vi "Img Load Frame Pic.vi"(8 "error in (no error)":errorcluster, 9 "Rectangle":T1, 10 "Image Path":path, 11 "Image In":T2) -> (0 "error out":errorcluster, 3 "Image Out":T2)   [LabVIEW 2018, in "Image Process.lvclass"]
uses:
  Image Process.lvclass
  <vilib>/vision/Image Controls.llb/IMAQ Image.ctl
panel:
  in  "threshold":u8=10
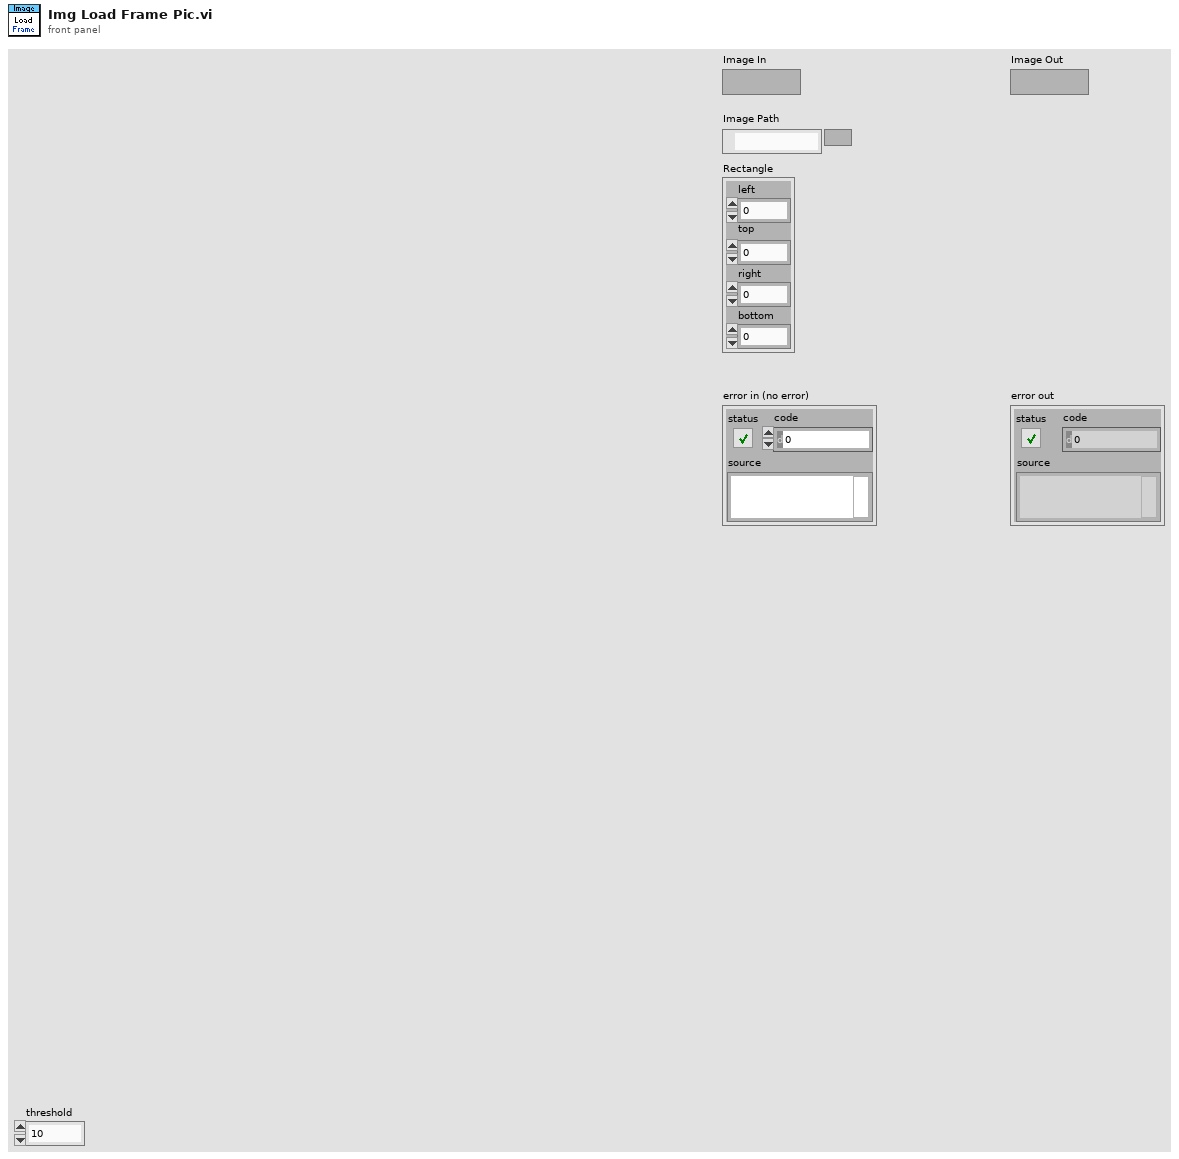
[diagram p1: front panel]
types:
  T1 = cluster{"left":i16, "top":i16, "right":i16, "bottom":i16}
  T2 = typedef "IMAQ Image.ctl" = refnum<image>
  T3 = typedef "imagedata.ctl" = cluster{"image type":i32, "image depth":i32, "image":u8[], "mask":u8[], "colors":u32[], "Rectangle":cluster{"left":i16, "top":i16, "right":i16, "bottom":i16}}
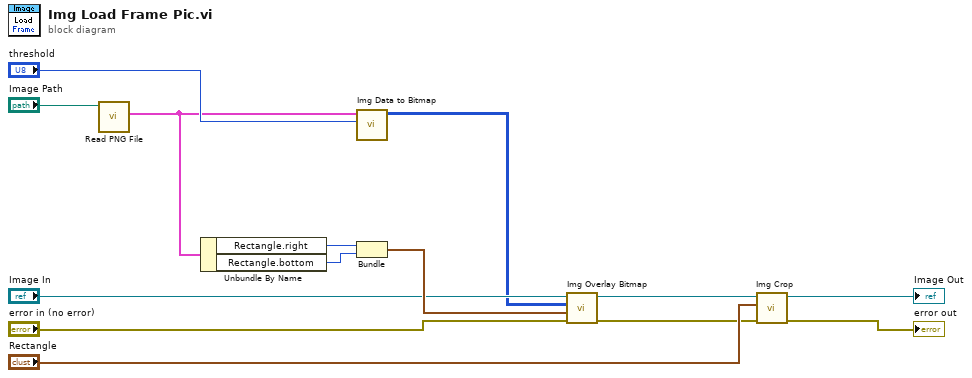
[diagram p0: block diagram]
diagram:
  n1 = call <vilib>:"Read PNG File.vi"("path to PNG file"="Image Path") -> ("image data"=w2:T3)  [unwired: 8 in, 2 out]
  n2 = Unbundle By Name(w2) -> ("Rectangle.right"=w14:i16, "Rectangle.bottom"=w13:i16)
  n3 = call "Img Data to Bitmap.vi"("threshold"="threshold", "image data"=w2) -> ("bitmap"=w1:u32[][])  [unwired: 8 in, 1 out]
  n4 = Bundle("right"=w14, "bottom"=w13) -> (w12:cluster{"right":i16, "bottom":i16})  [unwired: 1 in]
  n5 = call "Img Overlay Bitmap.vi"("error in (no error)"="error in (no error)", "Size"=w12, "Bitmap"=w1, "Image"="Image In") -> ("error out"=w4:errorcluster, "Image Out"=w11:T2)  [unwired: 6 in]
  n6 = call "Img Crop.vi"("error in (no error)"=w4, "Rectangle"="Rectangle", "Image Src"=w11) -> ("error out"=→"error out":errorcluster, "Image Out"=→"Image Out":T2)  [unwired: 7 in]
